vi "Create.vi"(8 "Error In":errorcluster, 11 "reference in":refnum<class "TraceWindow.lvclass">) -> (0 "Error Out":errorcluster, 3 "reference out":refnum<class "TraceWindow.lvclass">)   [LabVIEW 2021, in "TraceWindow.lvlib" / "TraceWindow.lvclass"]
uses:
  TraceWindow.lvclass
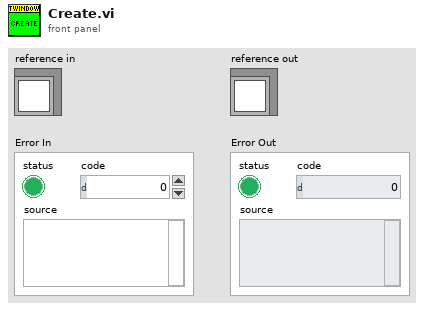
[diagram p1: front panel]
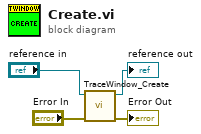
[diagram p0: block diagram]
diagram:
  n1 = call "TraceWindow_Create.vi"("Error In"="Error In", "reference in"="reference in") -> ("Error Out"=→"Error Out":errorcluster, "reference out"=→"reference out":refnum<class "TraceWindow.lvclass">)  [unwired: 8 in]
